vi "Intake Rotation Globals.vi"() -> ()   [LabVIEW 2017]
uses:
  Intake Rotation Notifier.ctl
panel:
  in  "Rotation Position":i32
  out "Intake Rotation Upper Limit Switch":bool
  in  "Intake Rotation Cals":dbl[](array[numeric])
  out "Intake Rotation Lower Limit Switch":bool
  in  "Intake Rotation Execute Notifier":refnum<notifier>
  in  "Intake Rotation Set Notifier":refnum<notifier>
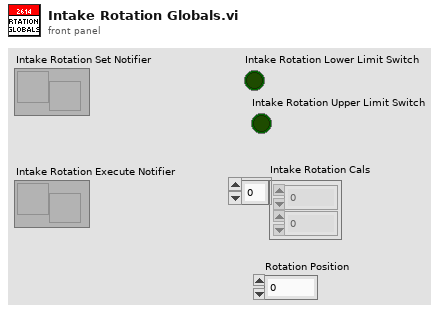
[diagram p1: front panel]
diagram:
